vi "VISAWriteWithEchoback.vi"(8 "error in":errorcluster, 9 "termination":string, 10 "write data":string, 11 "VISA resource name":refnum<visa-resource-name>) -> (0 "error out":errorcluster, 2 "written data":string, 3 "VISA resource name out":refnum<visa-resource-name>)   [LabVIEW 2020]
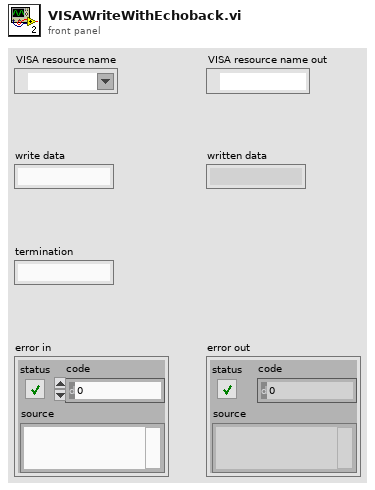
[diagram p1: front panel]
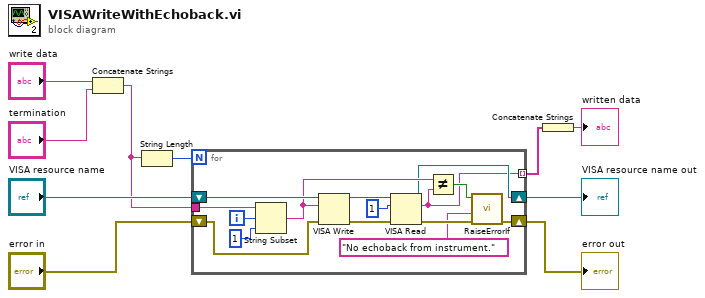
[diagram p0: block diagram]
diagram:
  n1 = Concatenate Strings("write data", "termination") -> (w5:string)
  n2 = String Length(string=w5) -> (length=w9:i32)
  n3 = for {
    N: w9 -> [_]
    tunnel: w5 -> [w20]
    shift-right: [w14] -> w6
    shift-left: "error in" -> [w13]
    shift-right: [w12] -> w3
    shift-left: "VISA resource name" -> [w21]
    tunnel: [w11] -> w2 mode=indexing
    i -> [w19]
    n4 = String Subset(string=w20, offset (0)=w19, length (rest)=1 ("length (rest)")) -> (substring=w15:string)
    n5 = VISA Write(VISA resource name=w21, write buffer=w15, error in (no error)=w13) -> (VISA resource name out=w25:refnum<visa-resource-name>, error out=w24:errorcluster)  [unwired: 1 out]
    n6 = VISA Read(VISA resource name=w25, byte count=u32 1, error in (no error)=w24) -> (VISA resource name out=w12:refnum<visa-resource-name>, read buffer=w11:string, error out=w23:errorcluster)  [unwired: 1 out]
    n7 = Not Equal?(x=w15, y=w11) -> (x != y?=w22:bool)
    n8 = call "RaiseErrorIf.vi"("error in (no error)"=w23, "error message"="No echoback from instrument.", "error? (true)"=w22) -> ("error out"=w14:errorcluster)  [unwired: 8 in]
  }
  "error out" <- w6
  "VISA resource name out" <- w3
  n9 = Concatenate Strings(w2) -> (→"written data":string)
